vi "close.vi"(8 "error in (no error)":errorcluster, 11 "data passing":T1) -> (0 "error out":errorcluster, 3 "data passing out":T1)   [LabVIEW 2016]
uses:
  data.ctl
  device.ctl
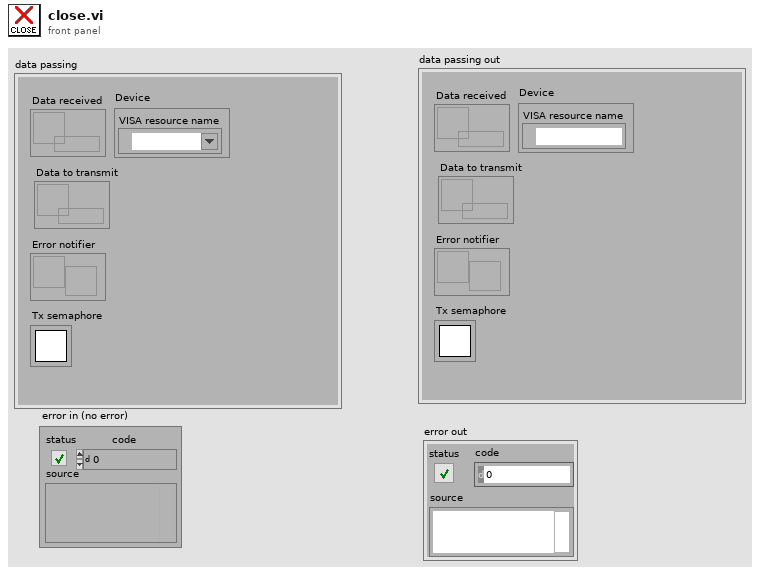
[diagram p1: front panel]
types:
  T1 = typedef "data.ctl" = cluster{"Data received":refnum<queue>, "Data to transmit":refnum<queue>, "Error notifier":refnum<notifier>, "Tx semaphore":T2, "Device":T3}
  T2 = typedef "Semaphore RefNum" = refnum<k1>
  T3 = typedef "device.ctl" = cluster{"VISA resource name":refnum<visa-resource-name>}
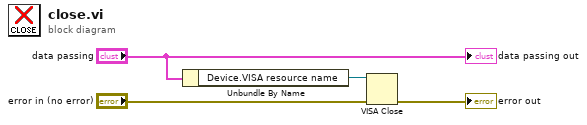
[diagram p0: block diagram]
diagram:
  n1 = Unbundle By Name("data passing") -> ("Device.VISA resource name"=w2:refnum<visa-resource-name>)
  n2 = VISA Close(VISA resource name=w2, error in (no error)="error in (no error)") -> (error out=→"error out":errorcluster)
  "data passing out" <- "data passing"
